vi "thcd_set_zrfs.vi"(4 "thcd_com":enum16{"Zero", "FullScale"}(ring), 5 "thcd_delay":u32=500, 6 "err_in":errorcluster, 8 "thcd_ch":T1, 9 "thcd_visa":refnum<visa-resource-name>) -> (0 "err_out":errorcluster, 1 "thcd_st":bool, 2 "thcd_res_msg":string, 3 "thcd_visa":refnum<visa-resource-name>)   [LabVIEW 2019]
uses:
  thcd_controls/ctrl_chn_thcd.ctl
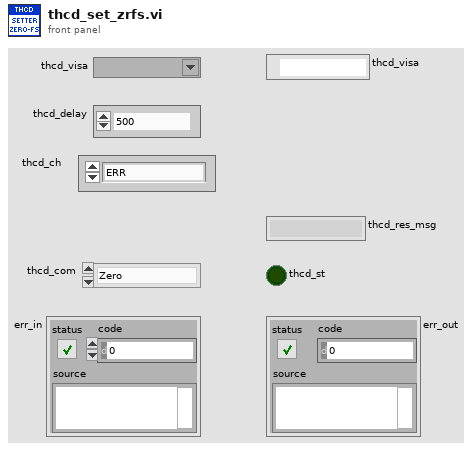
[diagram p1: front panel]
types:
  T1 = typedef "ctrl_chn_thcd.ctl" = enum8{"ERR", "1", "2", "3", "4"}
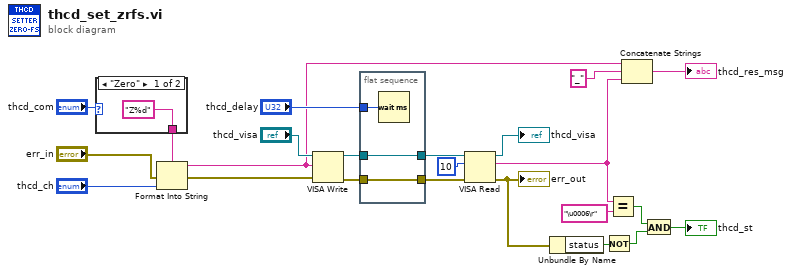
[diagram p0: block diagram]
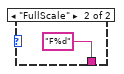
[diagram p2: hidden frame]
diagram:
  n1 = case shown="\"Zero\"" "thcd_com" {
    tunnel: ["Z%d" ("format string") "F%d" ("format string")] -> w17
    frame "Zero" {
    }
    frame "FullScale" {
    }
  }
  n2 = Format Into String(format string=w17, error in="err_in", "thcd_ch") -> (resulting string=w7:string, error out=w15:errorcluster)  [unwired: 1 in]
  n3 = VISA Write(VISA resource name="thcd_visa", write buffer=w7, error in (no error)=w15) -> (VISA resource name out=w22:refnum<visa-resource-name>, error out=w23:errorcluster)  [unwired: 1 out]
  n4 = flat-sequence {
    tunnel: w23 -> [w27]
    tunnel: [w27] -> w3
    tunnel: w22 -> [w26]
    tunnel: [w26] -> w4
    tunnel: "thcd_delay" -> [w28]
    frame #0 {
      n5 = Wait (ms)(milliseconds to wait=w28) -> ()  [unwired: 1 out]
    }
  }
  n6 = VISA Read(VISA resource name=w4, byte count=u32 10, error in (no error)=w3) -> (VISA resource name out=→"thcd_visa":refnum<visa-resource-name>, read buffer=w8:string, error out=w1:errorcluster)  [unwired: 1 out]
  "err_out" <- w1
  n7 = Unbundle By Name(w1) -> ("status"=w14:bool)
  n8 = Not(x=w14) -> (.not. x?=w11:bool)
  n9 = Equal?(x=w8, y="\u0006\r") -> (x = y?=w12:bool)
  n10 = Concatenate Strings(w7, "_", w8) -> (→"thcd_res_msg":string)
  n11 = And(x=w12, y=w11) -> (x .and. y?=→"thcd_st":bool)
